vi "getTemperature.vi"(6 "Channel":i32, 8 "error in (no error)":errorcluster, 11 "Instrument.TC.MNK in":refnum<class "Inst.TC.CF.lvclass">) -> (0 "error out":errorcluster, 1 "Status":string, 2 "Temperature (K)":dbl, 3 "Instrument.TC.MNK out":refnum<class "Inst.TC.CF.lvclass">, 4 "Finished?":bool)   [LabVIEW 2019, in "Inst.TC.CF.lvclass"]
uses:
  Inst.TC.CF.lvclass
  Inst.TC/Inst.TC.lvclass
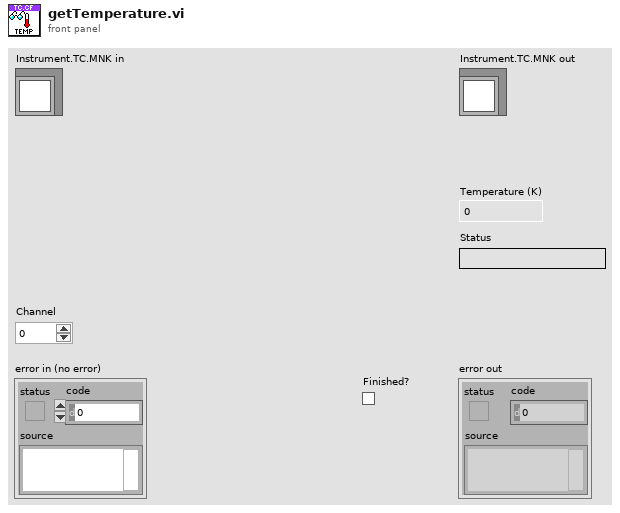
[diagram p1: front panel]
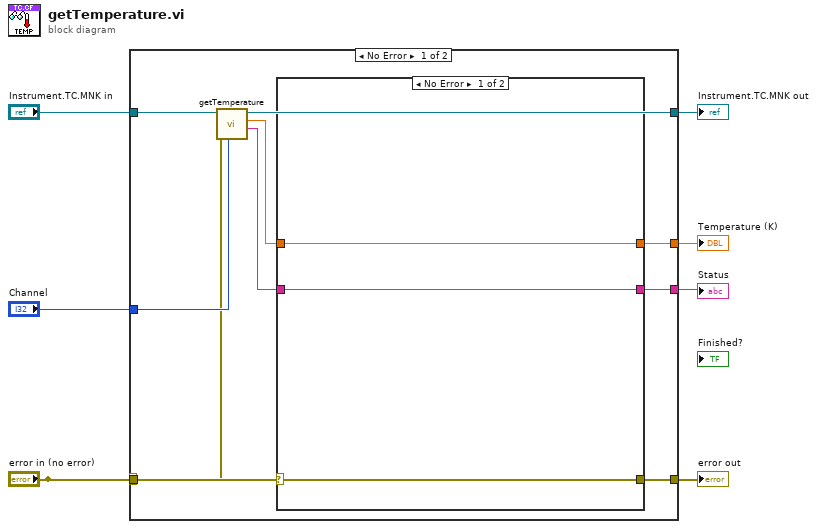
[diagram p0: block diagram]
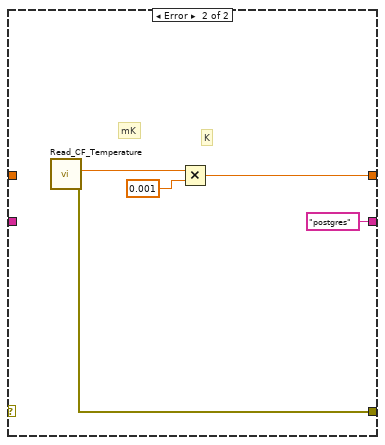
[diagram p2: hidden frame]
diagram:
  n1 = case shown="No Error" "error in (no error)" {
    selector: "error in (no error)" -> [w15 w26]
    tunnel: [w17 w26] -> w7
    tunnel: [w12 w27] -> w6
    tunnel: "Instrument.TC.MNK in" -> [w11 w27]
    tunnel: [w16 _] -> w4
    tunnel: "Channel" -> [w14 _]
    tunnel: "error in (no error)" -> [w13 _]
    tunnel: [w9 _] -> w1
    frame No Error {
      n2 = call-parent "getTemperature.vi"("Channel"=w14, "error in (no error)"=w13, "Inst.TC in"=w11) -> ("Status"=w8:string, "Temperature (K)"=w10:dbl, "Inst.TC out"=w12:refnum<class "Inst.TC.CF.lvclass">)  [unwired: 4 in, 2 out]
      n3 = case shown="No Error" w15 {
        selector: w15 -> [w18 _]
        tunnel: [w18 w24] -> w17
        tunnel: [w20 w22] -> w16
        tunnel: w10 -> [w20 _]
        tunnel: [w19 "postgres" ("Status")] -> w9
        tunnel: w8 -> [w19 _]
        frame No Error {
        }
        frame Error {
          # "K"
          # "mK"
          n4 = call "Read_CF_Temperature.vi"() -> ("Error out"=w24:errorcluster, "Temperature (mK)"=w25:dbl)  [unwired: 10 in]
          n5 = Multiply(x=w25, y=0.001) -> (x*y=w22:dbl)
        }
      }
    }
    frame Error {
    }
  }
  "error out" <- w7
  "Instrument.TC.MNK out" <- w6
  "Temperature (K)" <- w4
  "Status" <- w1
